vi "Shooter Speed Control.vi"(10 "Shooter Wheel PID gains":T1={"proportional gain (Kc)"=0.03, "integral time (Ti, min)"=0.0, "derivative time (Td, min)"=0.0} {"derivative time (Td, min)" format="%.3f"; "integral time (Ti, min)" format="%.3f"; "proportional gain (Kc)" format="%.3f"}, 11 "RPM wanted":dbl=1812.0) -> (1 "Current RPM":dbl, 2 "Spun Up":bool, 3 "Shooter Output":dbl=-0.0, 4 "Period (sec)":dbl=inf)   [LabVIEW 2013]
uses:
  <vilib>/Rock Robotics/WPI/Joystick/WPI_JoystickGetSetRefNum.vi
  Robot Global Data.vi
  Globals/Log Data.vi
  Globals/Useful Values.vi
  <vilib>/addons/control/pid/pid.llb/PID (DBL).vi
  <vilib>/addons/control/pid/NI_PID_pid.lvlib
panel:
  out "Waveform Chart":dbl(graph)
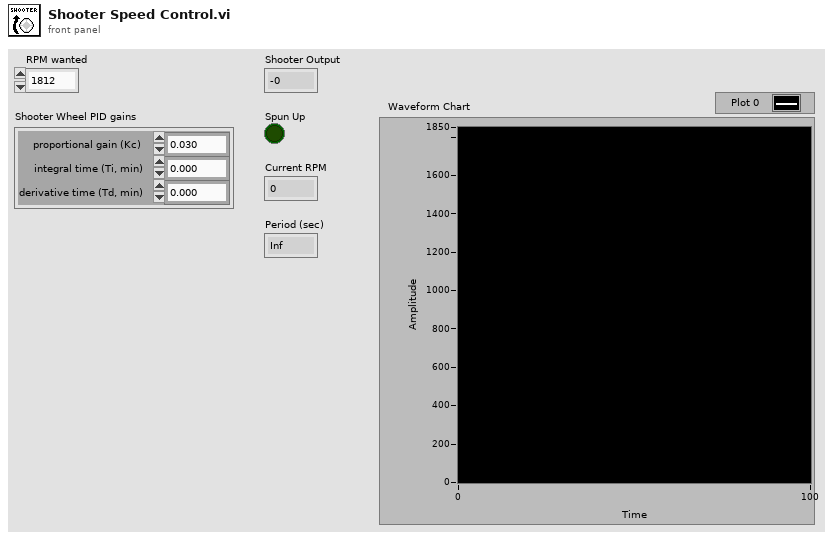
[diagram p1: front panel]
types:
  T1 = cluster{"proportional gain (Kc)":dbl, "integral time (Ti, min)":dbl, "derivative time (Td, min)":dbl}
  T2 = typedef "WPI_JoystickDevRef.ctl" = cluster{"Device":T3}
  T3 = typedef "WPI_JoystickDeviceEnum.ctl" = enum16{"USB 1", "USB 2", "USB 3", "USB 4", "Kinect 1", "Kinect 2"}
  T4 = typedef "WPI_MotorControlDeviceRef.ctl" = cluster{"DeviceStatus":errorcluster, "Type":enum16{"PWM", "CAN"}, "PWM":cluster{"Digital Module":T5, "PWM Channel":T6, "DeadBand":T7}, "CAN":cluster{"Device Number":u8, "Control Mode":T8, "Semaphore":T9, "Max Vout":dbl}, "Invert":bool, "TransformRef":T10, "InvTransformRef":T10}
  T5 = typedef "FPGA_TypedefDigitalModule.ctl" = enum16{"Digital Module 1", "Digital Module 2"}
  T6 = typedef "FPGA_DIOPWMChannel.ctl" = enum8{"PWM 1", "PWM 2", "PWM 3", "PWM 4", "PWM 5", "PWM 6", "PWM 7", "PWM 8", "PWM 9", "PWM 10", "Invalid"}
  T7 = typedef "WPI_PWMDeadband.ctl" = cluster{"Name":string, "maxPositivePwm":i32, "minPositivePwm":i32, "centerPwm":i32, "maxNegativePwm":i32, "minNegativePwm":i32, "angularRange":u16}
  T8 = typedef "WPI_CANJaguar_ControlMode.ctl" = enum8{"Percent VBus", "Current", "Speed", "Position", "Voltage"}
  T9 = typedef "Semaphore RefNum" = refnum<k1>
  T10 = typedef "WPI_PWMTransform_ConPane.ctl" = refnum<vi>
  T11 = typedef "WPI_CounterDevRef.ctl" = cluster{"DevStatus":errorcluster, "CntIndex":T12}
  T12 = typedef "FPGA_CounterCtrSystemIndex.ctl" = enum8{"Ctr 0", "Ctr 1", "Ctr 2", "Ctr 3", "Ctr 4", "Ctr 5", "Ctr 6", "Ctr 7", "Invalid"}
  T13 = typedef "WPI_JoystickButtonState.ctl" = cluster{"Button 1":bool, "Button 2":bool, "Button 3":bool, "Button 4":bool, "Button 5":bool, "Button 6":bool, "Button 7":bool, "Button 8":bool, "Button 9":bool, "Button 10":bool, "Button 11":bool, "Button 12":bool}
  T14 = typedef "WPI_DriverStationRobotMode2.ctl" = enum16{"Autonomous Disabled", "Autonomous Enabled", "Teleop Disabled", "Teleop Enabled", "Timeout", "Finish", "Test Disabled", "Test Enabled"}
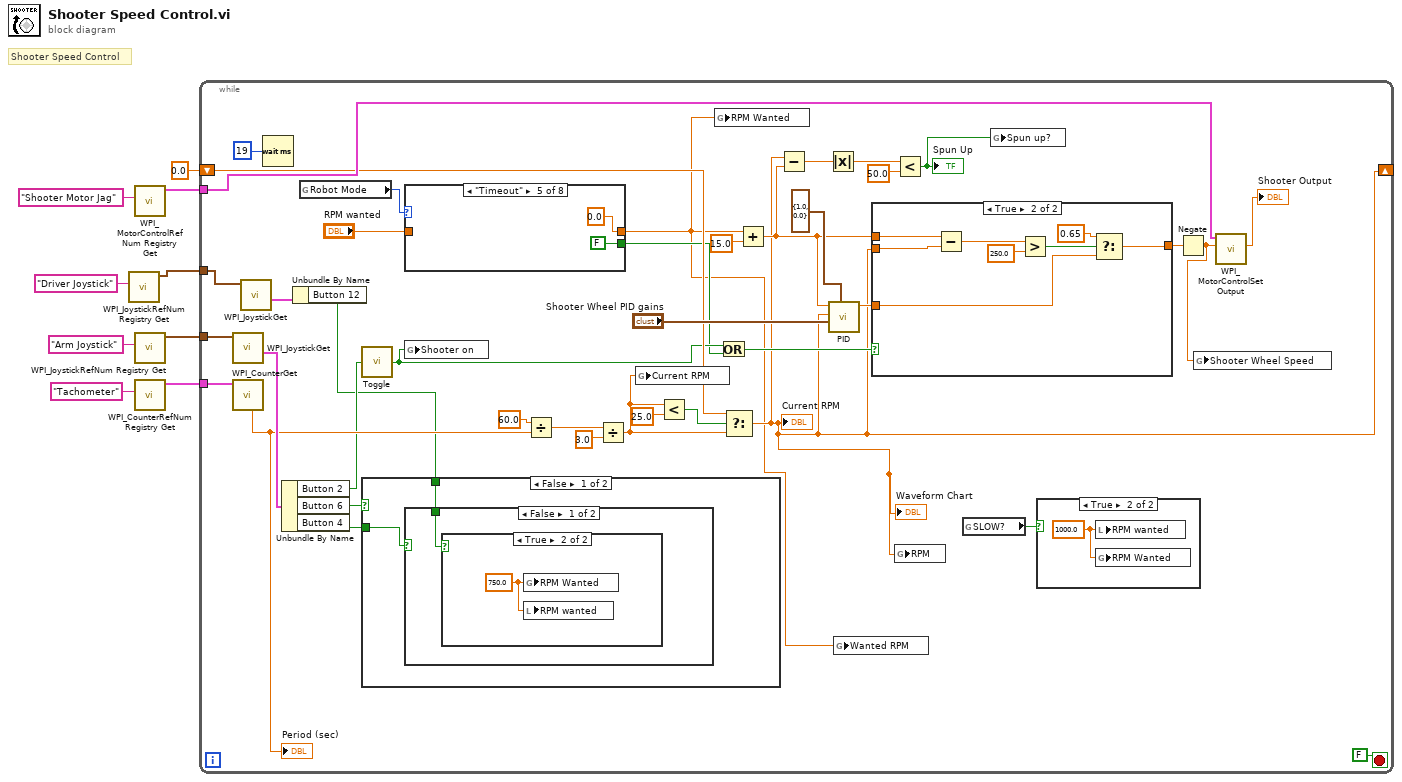
[diagram p0: block diagram]
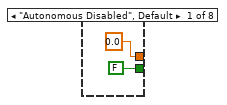
[diagram p3: hidden frame]
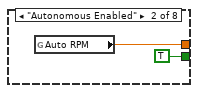
[diagram p4: hidden frame]
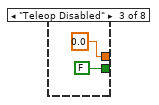
[diagram p5: hidden frame]
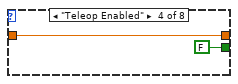
[diagram p6: hidden frame]
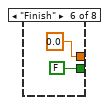
[diagram p7: hidden frame]
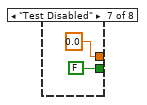
[diagram p8: hidden frame]
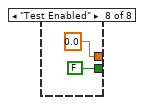
[diagram p9: hidden frame]
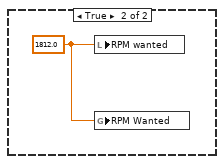
[diagram p11: hidden frame]
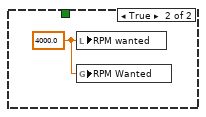
[diagram p12: hidden frame]
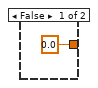
[diagram p13: hidden frame]
diagram:
  # "Shooter Speed Control"
  n1 = call <vilib>:"WPI_JoystickRefNum Registry Get.vi"("refnum name"="Driver Joystick") -> ("JoystickDevRef"=w1:T2)  [unwired: 9 in, 1 out]
  n2 = call <vilib>:"WPI_MotorControlRefNum Registry Get.vi"("refnum name"="Shooter Motor Jag") -> ("MotorControlDevRef"=w8:T4)  [unwired: 9 in, 1 out]
  n3 = call <vilib>:"WPI_JoystickRefNum Registry Get.vi"("refnum name"="Arm Joystick") -> ("JoystickDevRef"=w4:T2)  [unwired: 9 in, 1 out]
  n4 = call <vilib>:"WPI_CounterRefNum Registry Get.vi"("refnum name"="Tachometer") -> ("CounterDevRef"=w5:T11)  [unwired: 9 in, 1 out]
  n5 = while {
    tunnel: w4 -> [w47]
    tunnel: w5 -> [w41]
    tunnel: w8 -> [w39]
    shift-right: [w16] -> _
    shift-left: 0.0 -> [w36]
    tunnel: w1 -> [w13]
    stop <- FALSE stop-if-true
    n6 = call <vilib>:"WPI_JoystickGet.vi"("JoystickDevRef"=w47) -> ("Buttons"=w48:T13)  [unwired: 1 in, 5 out]
    n7 = call <vilib>:"WPI_CounterGet.vi"("CounterDevRef in"=w41) -> ("Period (sec)"=w43:dbl)  [unwired: 5 in, 5 out]
    "Period (sec)" <- w43
    n8 = call <vilib>:"WPI_JoystickGet.vi"("JoystickDevRef"=w13) -> ("Buttons"=w12:T13)  [unwired: 1 in, 5 out]
    n9 = Wait (ms)(milliseconds to wait=u32 19) -> ()  [unwired: 1 out]
    n10 = Unbundle By Name(w48) -> ("Button 2"=w32:bool, "Button 6"=w27:bool, "Button 4"=w26:bool)
    n11 = Unbundle By Name(w12) -> ("Button 12"=w11:bool)
    n12 = global read "Robot Global Data.vi" "Robot Mode"() -> (w22:T14)
    n13 = call "Toggle.vi"("Input"=w32) -> ("Output"=w23:bool)
    n14 = case shown="False" w27 {
      tunnel: w26 -> [w68 _]
      tunnel: w11 -> [w67 _]
      frame False {
        n15 = case shown="False" w68 {
          tunnel: w67 -> [w69 _]
          frame False {
            n16 = case shown="True" w69 {
              frame False {
              }
              frame True {
                w70 = 750.0 ("RPM wanted")
                n17 = global write "Useful Values.vi" "RPM Wanted"(w70) -> ()
                n18 = local write "RPM wanted"(w70) -> ()
              }
            }
          }
          frame True {
            w71 = 1812.0 ("RPM wanted")
            n19 = local write "RPM wanted"(w71) -> ()
            n20 = global write "Useful Values.vi" "RPM Wanted"(w71) -> ()
          }
        }
      }
      frame True {
        w72 = 4000.0 ("RPM wanted")
        n21 = local write "RPM wanted"(w72) -> ()
        n22 = global write "Useful Values.vi" "RPM Wanted"(w72) -> ()
      }
    }
    n23 = case shown="\"Timeout\"" w22 {
      tunnel: [0.0 ("RPM wanted") w54 0.0 ("RPM wanted") w58 0.0 ("RPM wanted") 0.0 ("RPM wanted") 0.0 ("RPM wanted") 0.0 ("RPM wanted")] -> w15
      tunnel: "RPM wanted" -> [_ _ _ w58 _ _ _ _]
      tunnel: [FALSE TRUE FALSE FALSE FALSE FALSE FALSE FALSE] -> w19
      frame "Autonomous Disabled", Default {
      }
      frame "Autonomous Enabled" {
        n24 = global read "Useful Values.vi" "Auto RPM"() -> (w54:dbl)
      }
      frame "Teleop Disabled" {
      }
      frame "Teleop Enabled" {
      }
      frame "Timeout" {
      }
      frame "Finish" {
      }
      frame "Test Disabled" {
      }
      frame "Test Enabled" {
      }
    }
    n25 = global write "Useful Values.vi" "Shooter on"(w23) -> ()
    n26 = Divide(x=60.0, y=w43) -> (x/y=w45:dbl)
    n27 = Divide(x=w45, y=3.0) -> (x/y=w17:dbl)
    n28 = global write "Useful Values.vi" "Current RPM"(w17) -> ()
    n29 = Less?(x=w17, y=25.0) -> (x < y?=w37:bool)
    n30 = global write "Useful Values.vi" "RPM Wanted"(w15) -> ()
    n31 = Or(x=w23, y=w19) -> (x .or. y?=w20:bool)
    n32 = Select(t=w36, s=w37, f=w17) -> (s? t:f=w16:dbl)
    "Current RPM" <- w16
    "Waveform Chart" <- w16
    n33 = Add(x=w15, y=15.0) -> (x+y=w25:dbl)
    n34 = Subtract(x=w16, y=w25) -> (x-y=w29:dbl)
    n35 = Absolute Value(x=w29) -> (abs(x)=w28:dbl)
    n36 = call-poly <vilib>:"PID.vi"("output range"=cluster{"output high":dbl, "output low":dbl} {"output high"=1.0, "output low"=0.0}, "PID gains"="Shooter Wheel PID gains", "process variable"=w16, "setpoint"=w25) -> ("output"=w34:dbl)  [unwired: 6 in, 1 out]
    n37 = global write "Log Data.vi" "Wanted RPM"(w15) -> ()
    n38 = case shown="True" w20 {
      tunnel: w25 -> [_ w77]
      tunnel: w16 -> [_ w76]
      tunnel: w34 -> [_ w79]
      tunnel: [0.0 ("output") w78] -> w33
      frame False {
      }
      frame True {
        n39 = Subtract(x=w77, y=w76) -> (x-y=w80:dbl)
        n40 = Greater?(x=w80, y=250.0) -> (0:w74:bool)
        n41 = Select(t=0.65, s=w74, f=w79) -> (s? t:f=w78:dbl)
      }
    }
    n42 = Less?(x=w28, y=50.0) -> (x < y?=w24:bool)
    "Spun Up" <- w24
    n43 = global write "Log Data.vi" "RPM"(w16) -> ()
    n44 = global read "Useful Values.vi" "SLOW?"() -> (w10:bool)
    n45 = global write "Useful Values.vi" "Spun up?"(w24) -> ()
    n46 = case shown="True" w10 {
      frame False {
      }
      frame True {
        w50 = 1000.0 ("RPM Wanted")
        n47 = local write "RPM wanted"(w50) -> ()
        n48 = global write "Useful Values.vi" "RPM Wanted"(w50) -> ()
      }
    }
    n49 = Negate(x=w33) -> (-x=w14:dbl)
    n50 = global write "Log Data.vi" "Shooter Wheel Speed"(w14) -> ()
    n51 = call <vilib>:"WPI_MotorControlSetOutput.vi"("Output"=w14, "MotorControlDevRef"=w39) -> ("Motor Output"=→"Shooter Output":dbl)  [unwired: 7 in, 2 out]
  }
